vi "ReceiverUI.vi"(11 "error in (no error)":errorcluster) -> (4 "Message Status":bool, 15 "error out":errorcluster)   [LabVIEW 2023, in "Receiver.lvclass"]
uses:
  Receiver.lvclass
  TypeDefs/ReceiverQueueOperations.ctl
  TypeDefs/ReceiverStateDataCluster.ctl
  TypeDefs/ReceiverDataCluster.ctl
  Communication/Communication.lvclass
  TypeDefs/UserEventOperations.ctl
  TypeDefs/SenderQueueOperations.ctl
  TypeDefs/SenderStateDataCluster.ctl
  Receiver.lvclass/Receiver.ctl
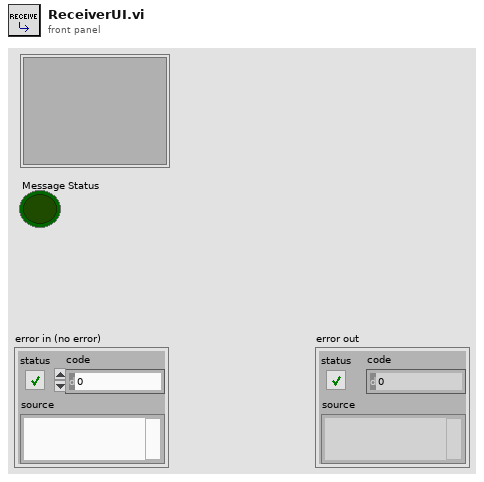
[diagram p1: front panel]
types:
  T1 = typedef "UserEventOperations.ctl" = enum16{"Create", "Generate", "Release"}
  T2 = typedef "ReceiverDataCluster.ctl" = cluster{"Received Data":variant, "Communicate Class":refnum<class "Communication.lvclass">, "Load Sender":bool, "Load Receiver":bool, "Run Sender":bool, "Receiver Class":refnum<class "Receiver.lvclass">, "Message Status":bool}
  T3 = typedef "ReceiverStateDataCluster.ctl" = cluster{"State":string, "Data":variant}
  T4 = typedef "ReceiverQueueOperations.ctl" = enum16{"Create", "Enqueue", "Dequeue", "Enqueue N", "Flush", "Close", "Enqueue N Stack"}
  T5 = typedef "SenderStateDataCluster.ctl" = cluster{"State":string, "Data":variant}
  T6 = typedef "SenderQueueOperations.ctl" = enum16{"Create", "Enqueue", "Dequeue", "Enqueue N", "Flush", "Close", "Enqueue N Stack"}
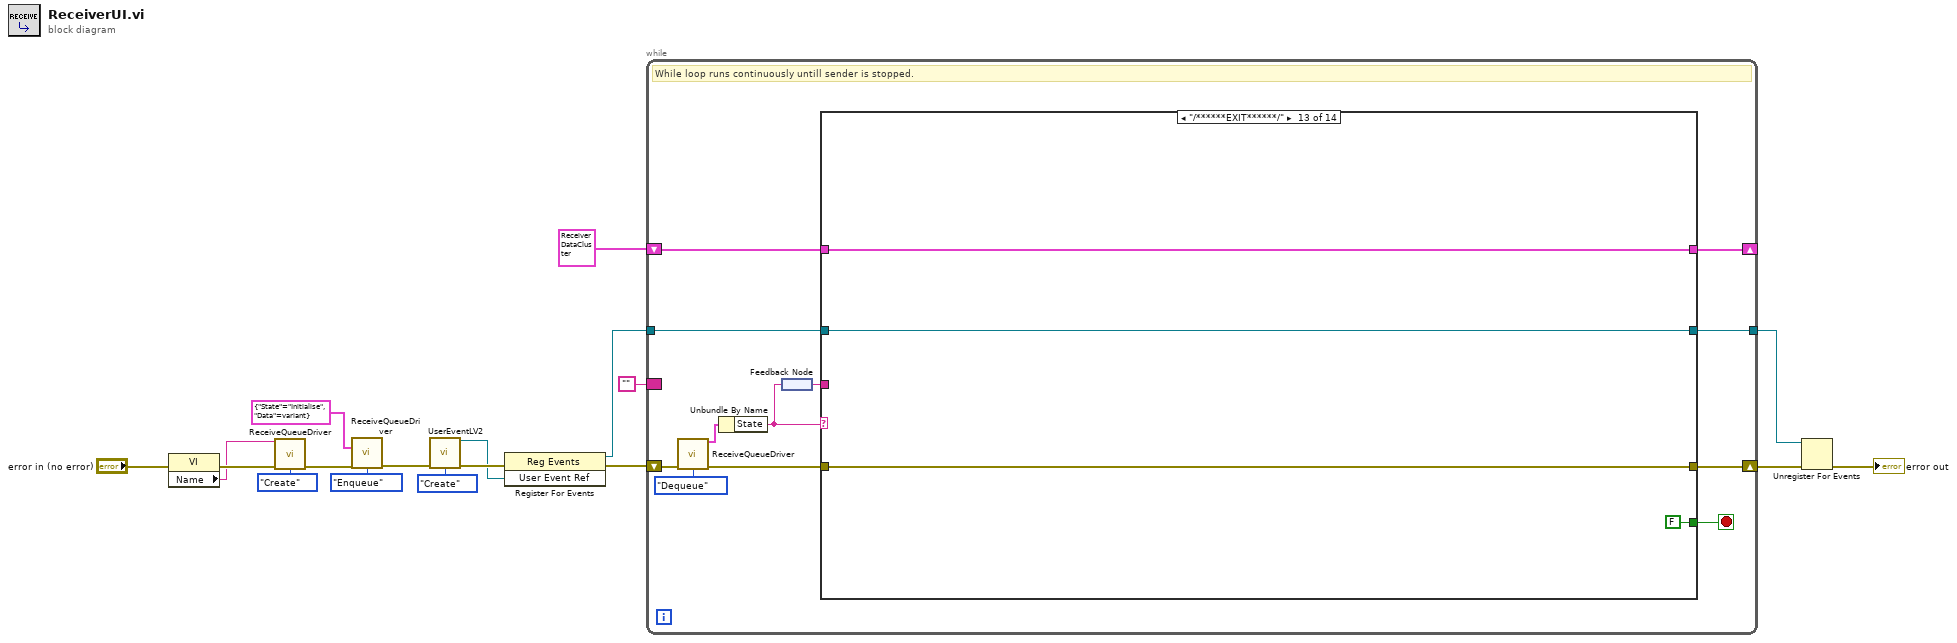
[diagram p0: block diagram]
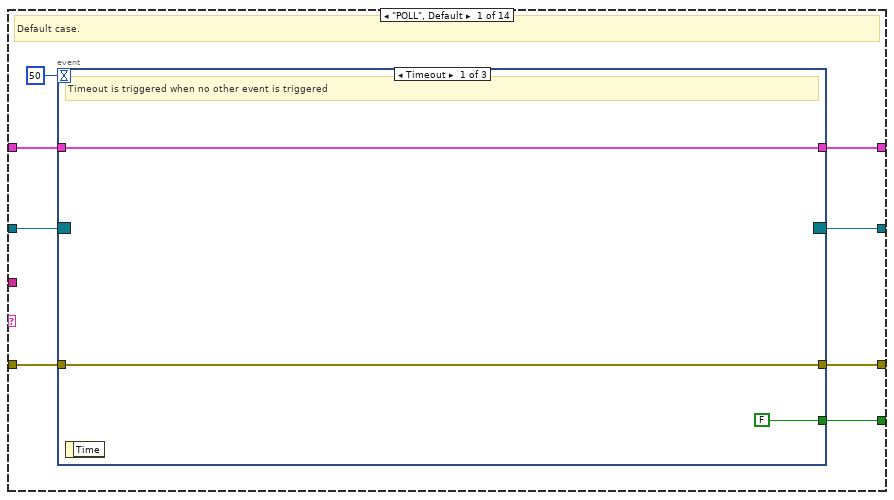
[diagram p2: hidden frame]
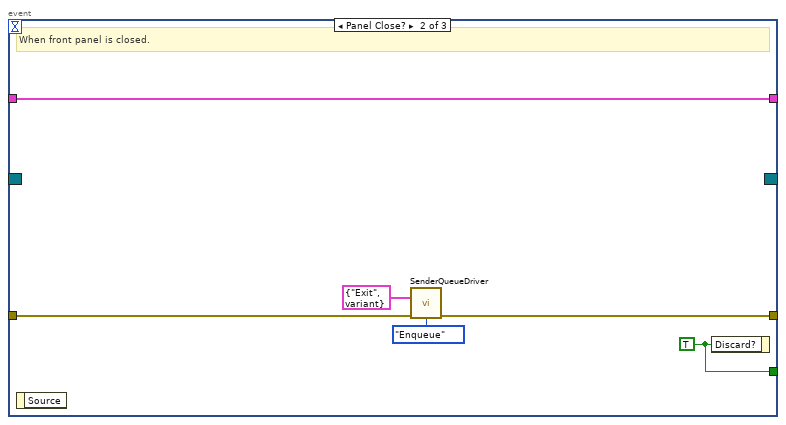
[diagram p3: hidden frame]
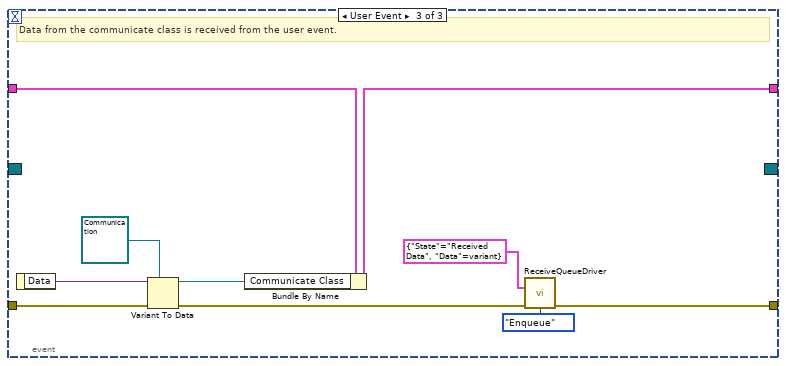
[diagram p4: hidden frame]
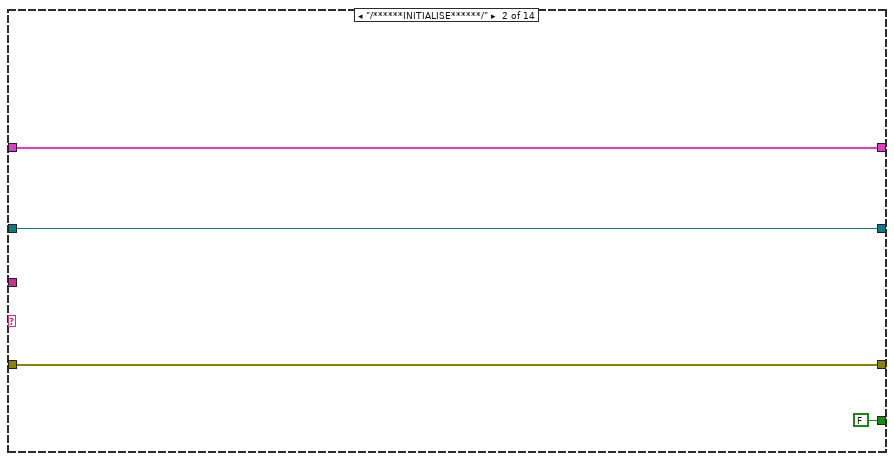
[diagram p5: hidden frame]
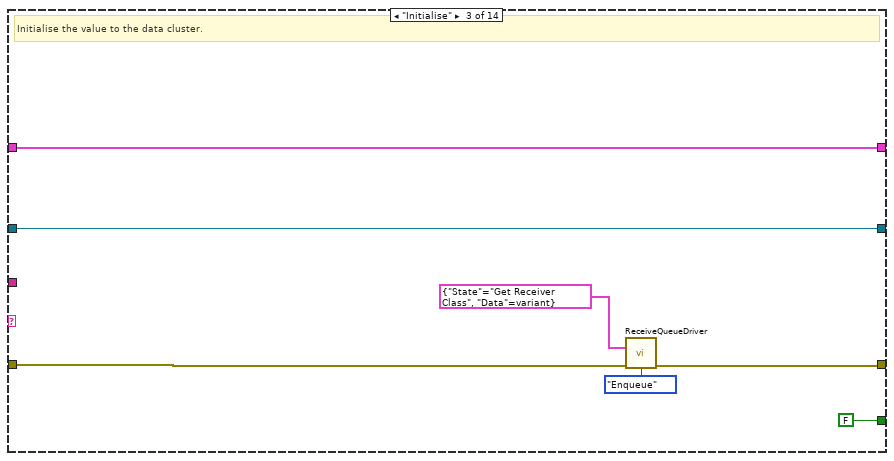
[diagram p6: hidden frame]
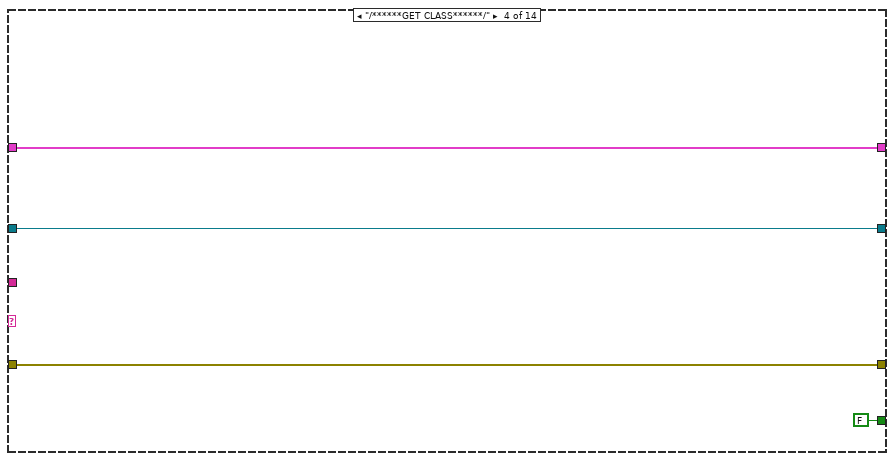
[diagram p7: hidden frame]
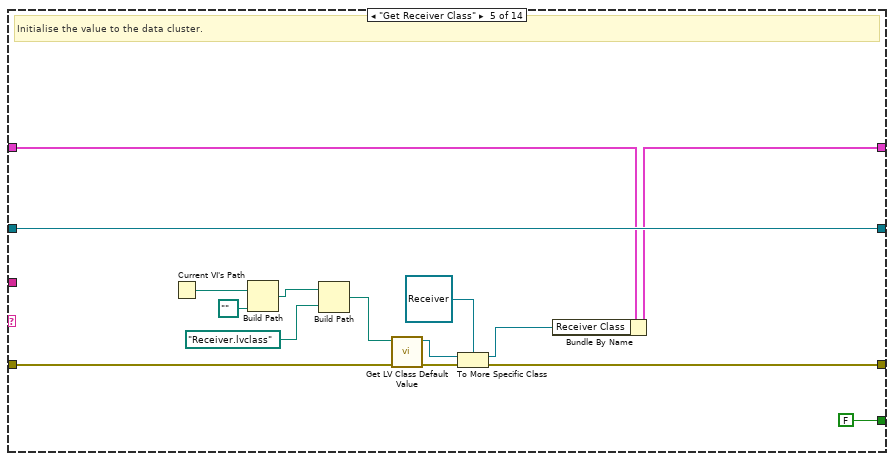
[diagram p8: hidden frame]
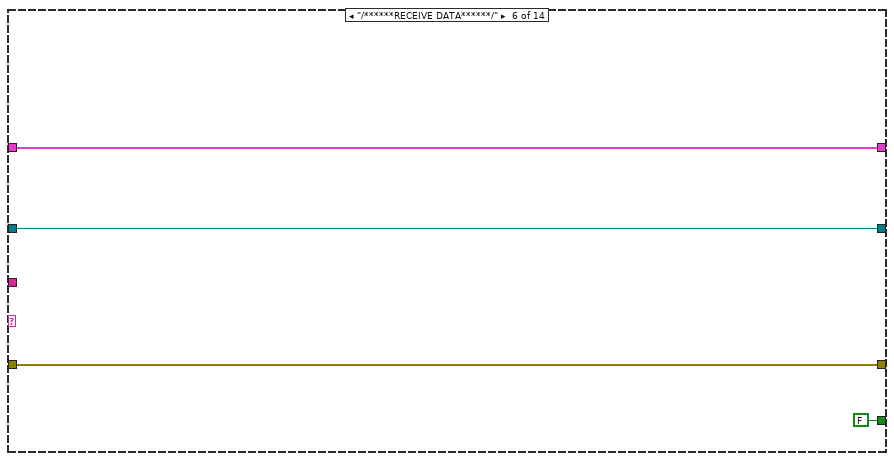
[diagram p9: hidden frame]
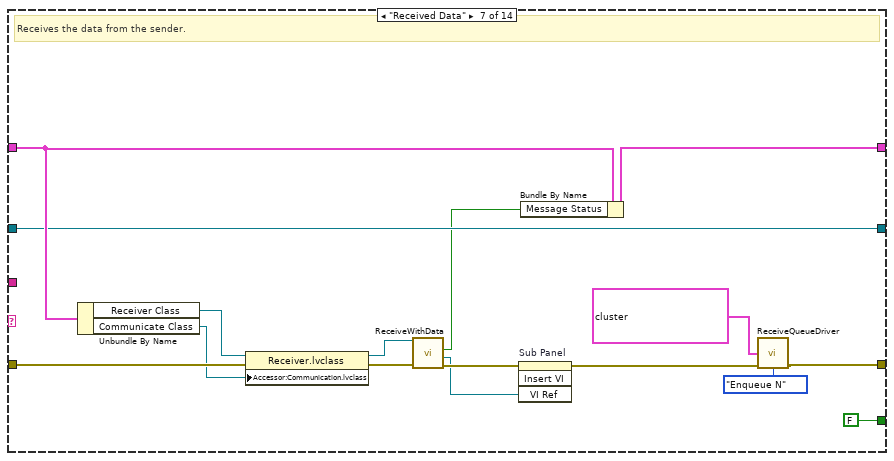
[diagram p10: hidden frame]
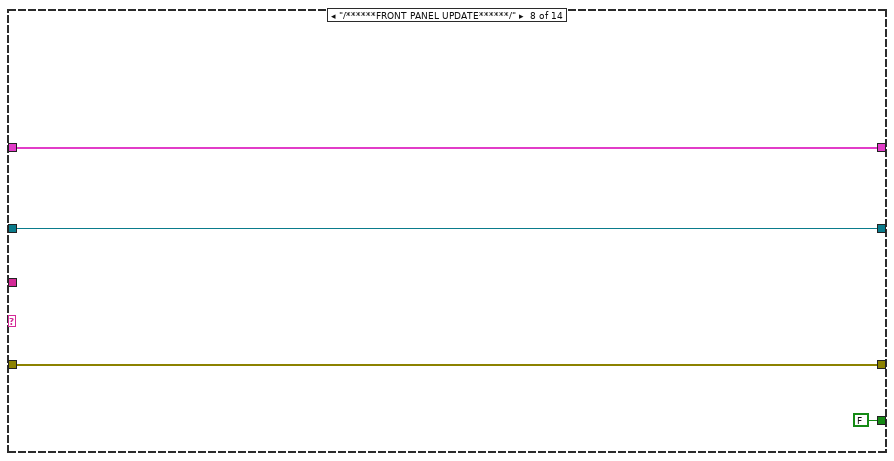
[diagram p11: hidden frame]
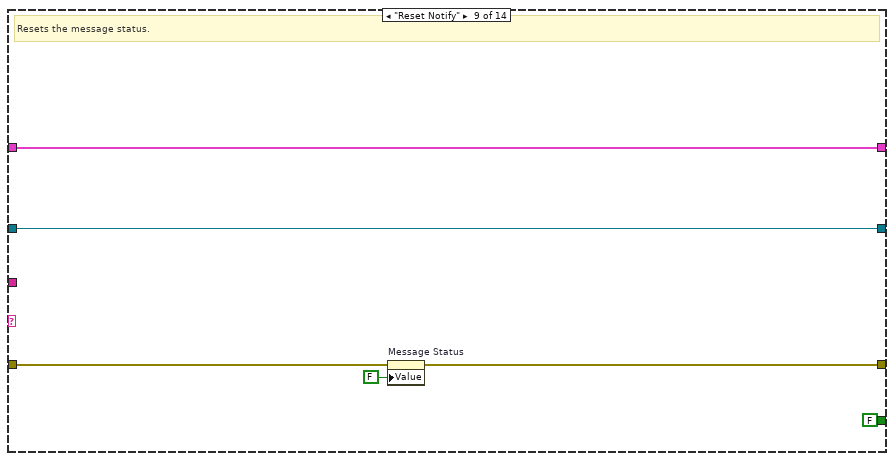
[diagram p12: hidden frame]
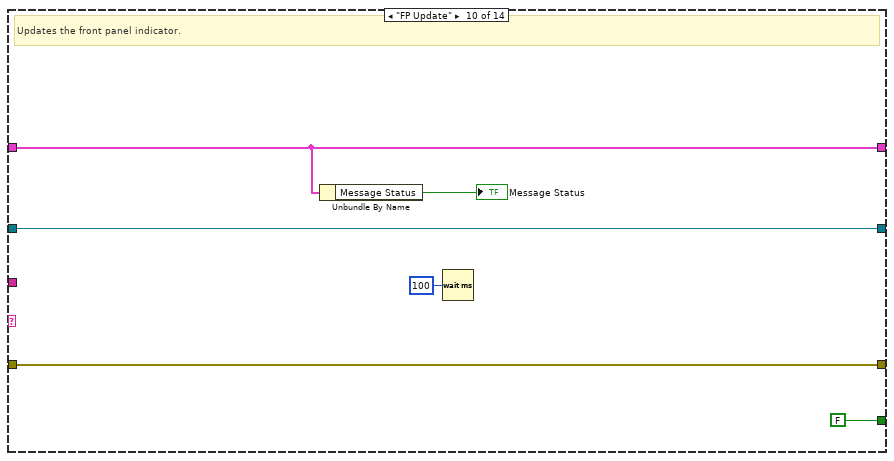
[diagram p13: hidden frame]
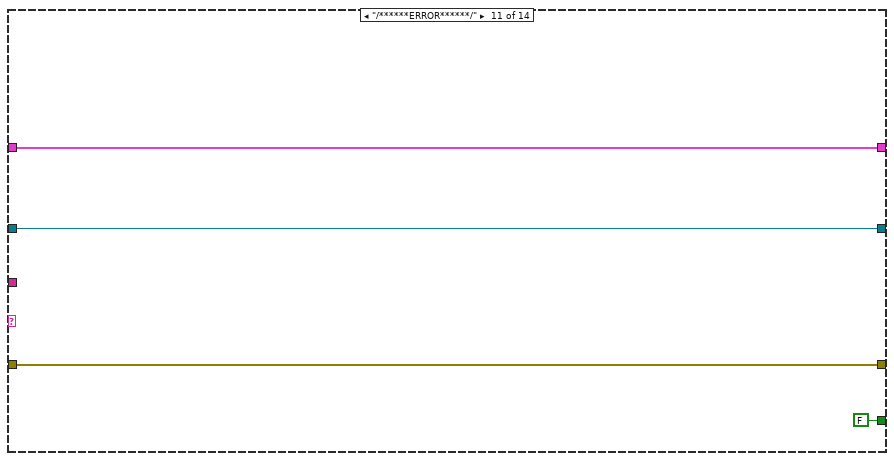
[diagram p14: hidden frame]
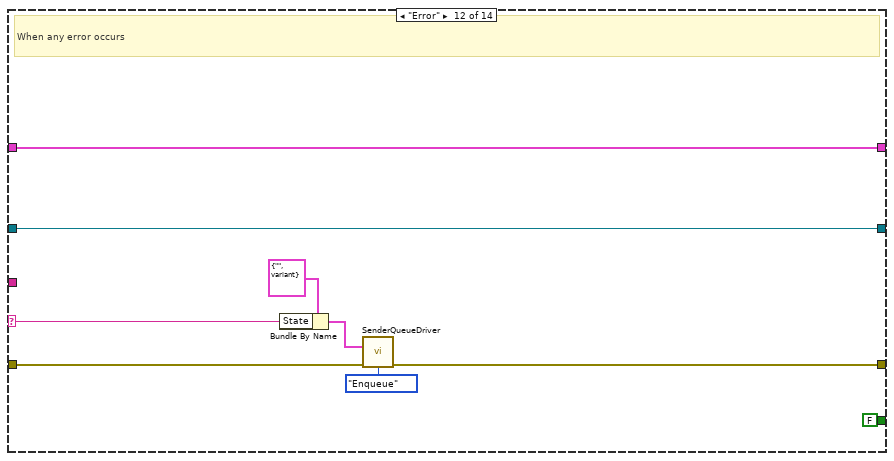
[diagram p15: hidden frame]
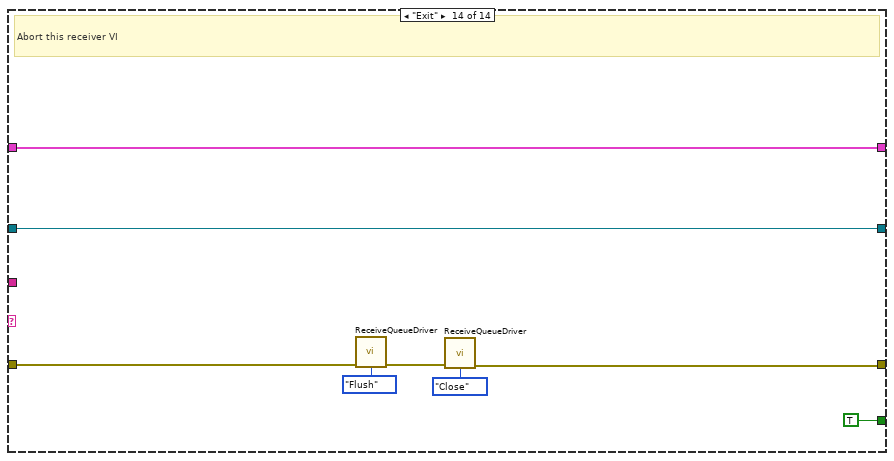
[diagram p16: hidden frame]
diagram:
  n1 = property class="VI"(error in="error in (no error)") -> (error out=w2:errorcluster, "Name"=w1:string)  [unwired: 1 in, 1 out]
  n2 = call "ReceiveQueueDriver.vi"("Queue Name"=w1, "error in (no error)"=w2, "Enum"=ReceiverQueueOperations."Create") -> ("error out"=w16:errorcluster)  [unwired: 11 in, 1 out]
  n3 = call "ReceiveQueueDriver.vi"("Enqueue Element"=T3 {"State"="Initialise", "Data"=variant}, "error in (no error)"=w16, "Enum"=ReceiverQueueOperations."Enqueue") -> ("error out"=w7:errorcluster)  [unwired: 11 in, 1 out]
  n4 = call "UserEventLV2.vi"("Error In"=w7, "Operation"=UserEventOperations."Create") -> ("User Event Ref"=w5:refnum<user-event>, "Error Out"=w6:errorcluster)  [unwired: 12 in]
  n5 = register-events(error in=w6, w5) -> (reference out=w9:refnum<event-registration>, error out=w10:errorcluster)  [unwired: 1 in]
  n6 = while {
    shift-right: [w30] -> w18
    shift-left: w10 -> [w29]
    shift-right: [w22] -> _
    shift-left: T2 {"Received Data"=variant, "Communicate Class"=refnum, "Load Sender"=FALSE, "Load Receiver"=FALSE, "Run Sender"=FALSE, "Receiver Class"=refnum, "Message Status"=FALSE} -> [w23]
    border: "" -> [_]
    tunnel: w9 -> [w20]
    tunnel: [w19] -> w3
    stop <- w26 stop-if-true
    # "While loop runs continuously untill sender is stopped."
    n7 = call "ReceiveQueueDriver.vi"("error in (no error)"=w29, "Enum"=ReceiverQueueOperations."Dequeue") -> ("Dequeue Element"=w27:T3, "error out"=w28:errorcluster)  [unwired: 12 in]
    n8 = Unbundle By Name(w27) -> ("State"=w25:string)
    n9 = feedback-in #1(w25) -> ()
    n10 = feedback #1() -> (w24:string)
    n11 = case shown="\"/******EXIT******/\"" w25 {
      selector: w25 -> [_ _ _ _ _ _ _ _ _ _ _ w129 _ _]
      tunnel: w28 -> [w37 w59 w65 w70 w76 w89 w104 w109 w117 w122 w125 w133 w138 w145]
      tunnel: [w36 w59 w64 w70 w75 w89 w99 w109 w113 w122 w125 w132 w138 w141] -> w30
      tunnel: [w38 FALSE ("Discard?") FALSE FALSE ("Discard?") FALSE FALSE ("Discard?") FALSE FALSE ("Discard?") FALSE FALSE FALSE ("Discard?") FALSE FALSE ("Discard?") TRUE] -> w26
      tunnel: w24 -> [_ _ _ _ _ _ _ _ _ _ _ _ _ _]
      tunnel: w23 -> [w34 w61 w66 w72 w74 w91 w103 w111 w115 w120 w127 w136 w140 w148]
      tunnel: [w33 w61 w66 w72 w73 w91 w97 w111 w115 w120 w127 w136 w140 w148] -> w22
      tunnel: w20 -> [w32 w60 w67 w71 w86 w90 w101 w110 w116 w123 w126 w135 w139 w146]
      tunnel: [w31 w60 w67 w71 w86 w90 w101 w110 w116 w123 w126 w135 w139 w146] -> w19
      frame "POLL", Default {
        # "Default case."
        n12 = event shown="[0] Timeout" {
          selector: w32 -> [_ _ _]
          dyn-events: [_ _ _] -> w31
          timeout: 50 -> [_ _ _]
          tunnel: [FALSE w46 _] -> w38
          tunnel: w37 -> [w40 w45 w57]
          tunnel: [w40 w43 w49] -> w36
          tunnel: w34 -> [w39 w47 w56]
          tunnel: [w39 w47 w55] -> w33
          event Timeout {
            # "Timeout is triggered when no other event is triggered"
            n13 = event-data() -> ()  [unwired: 1 in, 1 out]
          }
          event Panel Close? {
            w46 = TRUE ("Discard?")
            # "When front panel is closed."
            n14 = event-data() -> ()  [unwired: 1 in, 1 out]
            n15 = call "SenderQueueDriver.vi"("Enqueue Element"=T5 {"State"="Exit", "Data"=variant}, "error in (no error)"=w45, "Enum"=SenderQueueOperations."Enqueue") -> ("error out"=w43:errorcluster)  [unwired: 11 in, 1 out]
            n16 = event-data("Discard?"=w46) -> ()  [unwired: 1 in, 1 out]
          }
          event User Event {
            # "Data from the communicate class is received from the user event."
            n17 = event-data() -> ("Data"=w54:variant)  [unwired: 1 in]
            n18 = Variant To Data(error in=w57, type=refnum<class "Communication.lvclass"> refnum ("Communicate Class"), Variant=w54) -> (data=w52:refnum<class "Communication.lvclass">, error out=w50:errorcluster)
            n19 = Bundle By Name(cluster=w56, "Communicate Class"=w52) -> (w55:T2)
            n20 = call "ReceiveQueueDriver.vi"("Enqueue Element"=T3 {"State"="Received Data", "Data"=variant}, "error in (no error)"=w50, "Enum"=ReceiverQueueOperations."Enqueue") -> ("error out"=w49:errorcluster)  [unwired: 11 in, 1 out]
          }
        }
      }
      frame "/******INITIALISE******/" {
      }
      frame "Initialise" {
        # "Initialise the value to the data cluster."
        n21 = call "ReceiveQueueDriver.vi"("Enqueue Element"=T3 {"State"="Get Receiver Class", "Data"=variant}, "error in (no error)"=w65, "Enum"=ReceiverQueueOperations."Enqueue") -> ("error out"=w64:errorcluster)  [unwired: 11 in, 1 out]
      }
      frame "/******GET CLASS******/" {
      }
      frame "Get Receiver Class" {
        # "Initialise the value to the data cluster."
        n22 = Current VI's Path() -> (path=w85:path)
        n23 = Build Path(base path=w85, name or relative path=path "..") -> (appended path=w83:path)
        n24 = Build Path(base path=w83, name or relative path=path "Receiver.lvclass") -> (appended path=w80:path)
        n25 = call <vilib>:"Get LV Class Default Value.vi"("error in (no error)"=w76, "class path"=w80) -> ("error out"=w81:errorcluster, "object"=w79:refnum<class>)  [unwired: 8 in]
        n26 = To More Specific Class(target class=refnum<class "Receiver.lvclass"> refnum ("Receiver.lvclass"), reference=w79, error in=w81) -> (specific class reference=w77:refnum<class "Receiver.lvclass">, error out=w75:errorcluster)
        n27 = Bundle By Name(cluster=w74, "Receiver Class"=w77) -> (w73:T2)
      }
      frame "/******RECEIVE DATA******/" {
      }
      frame "Received Data" {
        # "Receives the data from the sender."
        n28 = Unbundle By Name(w103) -> ("Receiver Class"=w98:refnum<class "Receiver.lvclass">, "Communicate Class"=w102:refnum<class "Communication.lvclass">)
        n29 = property class="Receiver.lvclass"(reference=w98, error in=w104, "Accessor:Communication.lvclass"=w102) -> (reference out=w105:refnum<class "Receiver.lvclass">, error out=w106:errorcluster)
        n30 = call "ReceiveWithData.vi"("error in (no error)"=w106, "Receiver in"=w105) -> ("error out"=w95:errorcluster, "VI Ref"=w93:refnum<vi>, "Message Status"=w92:bool)  [unwired: 6 in, 1 out]
        n31 = invoke on="Sub Panel" class="SubPnl" method="Insert VI"(error in=w95, "VI Ref"=w93) -> (error out=w94:errorcluster)  [unwired: 2 in, 3 out]
        n32 = Bundle By Name(cluster=w103, "Message Status"=w92) -> (w97:T2)
        n33 = call "ReceiveQueueDriver.vi"("Enqueue N Element"=T3[] [{"State"="FP Update", "Data"=variant}, {"State"="Reset Notify", "Data"=variant}], "error in (no error)"=w94, "Enum"=ReceiverQueueOperations."Enqueue N") -> ("error out"=w99:errorcluster)  [unwired: 11 in, 1 out]
      }
      frame "/******FRONT PANEL UPDATE******/" {
      }
      frame "Reset Notify" {
        # "Resets the message status."
        n34 = property on="Message Status" class="Bool (strict)"(error in=w117, "Value"=FALSE ("Message Status")) -> (error out=w113:errorcluster)  [unwired: 1 in, 1 out]
      }
      frame "FP Update" {
        # "Updates the front panel indicator."
        n35 = Unbundle By Name(w120) -> ("Message Status"=→"Message Status":bool)
        n36 = Wait (ms)(milliseconds to wait=u32 100) -> ()  [unwired: 1 out]
      }
      frame "/******ERROR******/" {
      }
      frame "Error" {
        # "When any error occurs"
        n37 = Bundle By Name(cluster=T5 {"State"="", "Data"=variant} ("Enqueue Element"), "State"=w129) -> (w128:T5)
        n38 = call "SenderQueueDriver.vi"("Enqueue Element"=w128, "error in (no error)"=w133, "Enum"=SenderQueueOperations."Enqueue") -> ("error out"=w132:errorcluster)  [unwired: 11 in, 1 out]
      }
      frame "/******EXIT******/" {
      }
      frame "Exit" {
        # "Abort this receiver VI"
        n39 = call "ReceiveQueueDriver.vi"("error in (no error)"=w145, "Enum"=ReceiverQueueOperations."Flush") -> ("error out"=w144:errorcluster)  [unwired: 12 in, 1 out]
        n40 = call "ReceiveQueueDriver.vi"("error in (no error)"=w144, "Enum"=ReceiverQueueOperations."Close") -> ("error out"=w141:errorcluster)  [unwired: 12 in, 1 out]
      }
    }
  }
  n41 = Unregister For Events(event registration refnum=w3, error in=w18) -> (error out=→"error out":errorcluster)
